vi "SMTP Email No EOC Error.vi"(4 "error in (no error)":errorcluster) -> (1 "error out":errorcluster)   [LabVIEW 2011, in "NewNI_SMTPEmail.lvlib"]
doc: "No EOC Error.vi checks to see if a connection closed error occurred and resets it to no error."
uses:
  NewNI_SMTPEmail.lvlib
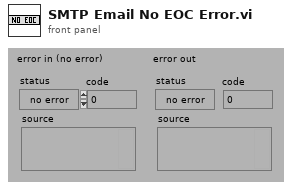
[diagram p1: front panel]
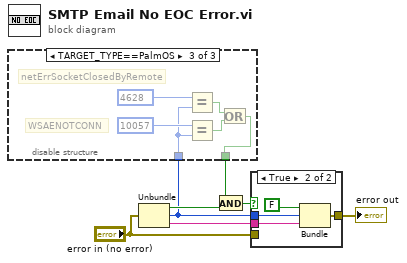
[diagram p0: block diagram]
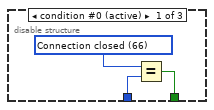
[diagram p2: hidden frame]
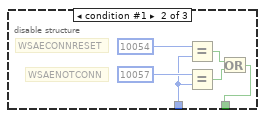
[diagram p3: hidden frame]
diagram:
  n1 = Unbundle("error in (no error)") -> ("status"=w6:bool, "code"=w2:i32, "source"=w3:string)
  n2 = disable-structure shown="TARGET_TYPE==PalmOS" {
    disable-tunnel: [w10 w11 w17] -> w5
    disable-tunnel: w2 -> [w9 w15 w21]
    frame condition #0 (active) {
      w8 = u16 66 items=["No Error", "Argument Error", "Memory Full", "Out of Zone", "End of File", "File Already Open", "Generic File IO Error", "File Not Found", "File Permission Error", "Disk Full", "Duplicate Path", "Too Many Files Open", "Not Enabled", "Resource File Not Found", "Cannot Add Resource", "Resource Not Found", "Image Not Found", "Image Memory Error", "Pen Does Not Exist", "Config Bad Type", "Config Token Not Found", "Config Parse Error", "Config Memory Error", "Bad External Code Format", "Bad External Code Offset", "External Code Not Present", "Null Window", "Destroy Window Mixup", "Null Menu", "Print Aborted", "Bad Print Record", "Print Driver Error", "Windows Error During Print", "Memory Error During Print", "Print Dialog Error", "Generic Print Error", "Invalid Device Refnum", "Device Not Found", "Device Parameter Error", "Device Unit Error", "Can't Open Device", "Device Call Aborted", "Generic Error", "Cancelled By User", "Object ID Too Low", "Object ID Too High", "Object Not In Heap", "Unknown Heap", "Bad DefProc ID", "DefProc Not In Table", "Message Out Of Range", "Null Method", "Unknown Message", "Manager Call Not Supported", "Bad address", "Connection In progress", "Connection timed out", "Connection is already in progress", "Network attribute not supported", "Network error", "Address in use", "System out of memory", "Connection aborted", "Connection refused", "Connection is not connected", "Connection is already connected", "Connection closed", "Initialize error (interapplication manager)", "Bad occurrence", "Wait on unbound occurrence handler", "Occurrence queue overflow", "Bad path", "Semaphore not signaled", "Unrecognized type (interapplication manager)"]
      n3 = Equal?(x=w8, y=w9) -> (x = y?=w10:bool)
    }
    frame condition #1 {
      # "WSAECONNRESET"
      # "WSAENOTCONN"
      n4 = Equal?(x=10054, y=w15) -> (x = y?=w13:bool)
      n5 = Equal?(x=10057, y=w15) -> (x = y?=w12:bool)
      n6 = Or(x=w13, y=w12) -> (x .or. y?=w11:bool)
    }
    frame condition #2 {
      # "netErrSocketClosedByRemote"
      # "WSAENOTCONN"
      n7 = Equal?(x=4628, y=w21) -> (x = y?=w19:bool)
      n8 = Equal?(x=10057, y=w21) -> (x = y?=w18:bool)
      n9 = Or(x=w19, y=w18) -> (x .or. y?=w17:bool)
    }
  }
  n10 = And(x=w5, y=w6) -> (x .and. y?=w4:bool)
  n11 = case shown="True" w4 {
    tunnel: "error in (no error)" -> [w23 _]
    tunnel: [w23 w27] -> w1
    tunnel: w3 -> [_ w26]
    tunnel: w2 -> [_ w25]
    frame False {
    }
    frame True {
      n12 = Bundle(FALSE, "code"=w25, "source"=w26) -> (w27:cluster{bool, "code":i32, "source":string})  [unwired: 1 out]
    }
  }
  "error out" <- w1
